vi "Actor Core.vi"(8 "error in":errorcluster, 11 "PRM in":refnum<class "PRM.lvclass">) -> (0 "error out":errorcluster, 3 "Actor out":refnum<class "Actor.lvclass">)   [LabVIEW 2019, in "PRM.lvlib" / "PRM.lvclass"]
doc: "The instrument actor core is only here to distribute panel resolution settings to children classes."
uses:
  Library/PRM.lvclass
  builds/Engine/Actor Framework.lvlibp/1abvi3w/vi.lib/ActorFramework/Actor/Actor.lvclass
  Custom Controls/Units.ctl
  PRM Messages/Set Channel by Name Msg/Set Channel by Name Msg.lvclass/Set Channel by Name Msg.ctl
  builds/Engine/Actor Framework.lvlibp/1abvi3w/vi.lib/ActorFramework/Message Enqueuer/Enqueue.vi
  PRM Messages/Set Channel by Name Msg/Set Channel by Name Msg.lvclass
  builds/Instruments/Instruments.lvlibp/Library/Instruments.lvclass
  C:/Users/Public/Documents/Development/builds/Instruments/Instruments.lvlibp/Library/Instruments.lvclass
panel:
  in  "Active Device":u16(ring)
  in  "Units":T1
  in  "Target":dbl caption="Ohms"
  in  "Active Channel":u16(ring) caption="Channel"
  in  "Apply":bool
  in  "Status":i32(listbox)
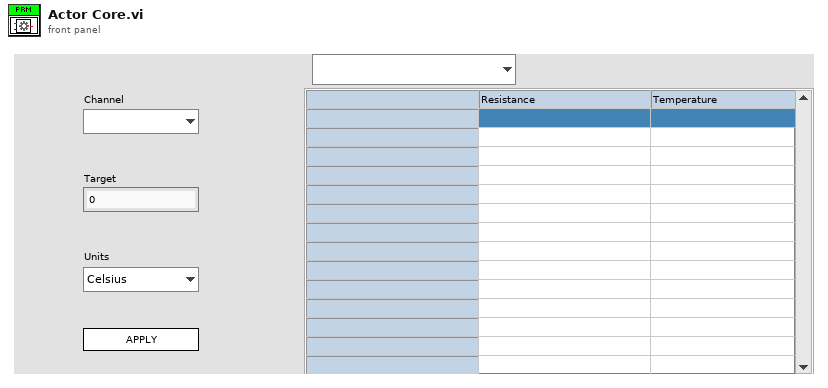
[diagram p1: front panel]
types:
  T1 = typedef "PRM.lvlib/PRM.lvclass/Units.ctl" = enum16{"Celsius", "Fahrenheit", "Kelvin", "Ohms"}
  T2 = cluster{"Pnl Actor":refnum<event-registration>, "Event Registration Refnum":refnum<event-registration>}
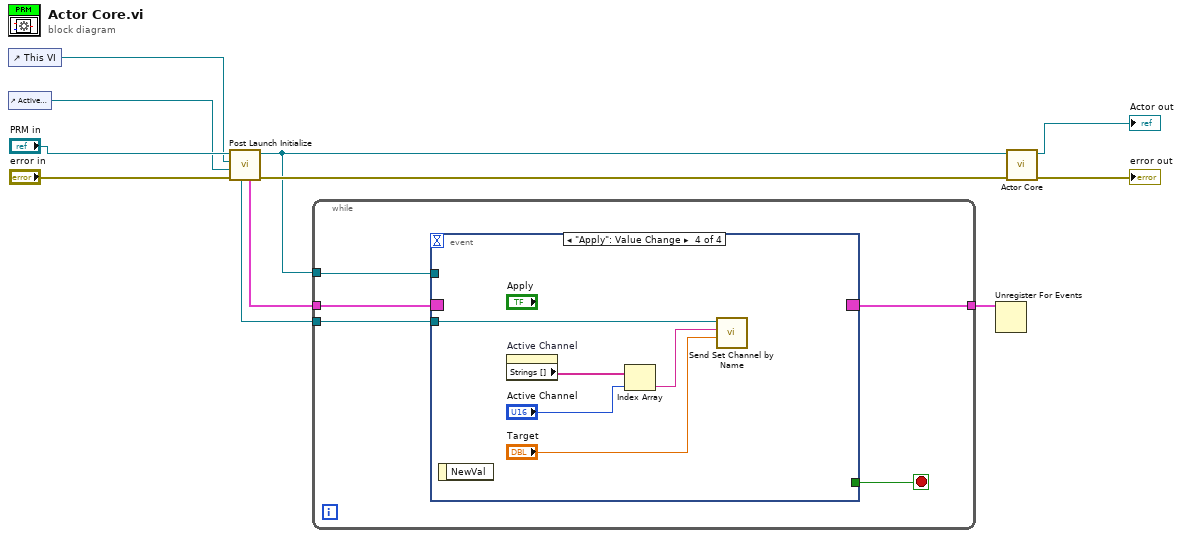
[diagram p0: block diagram]
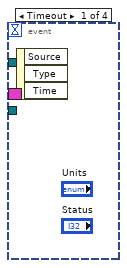
[diagram p2: hidden frame]
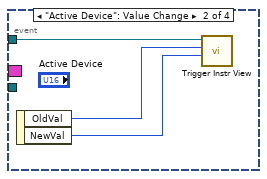
[diagram p3: hidden frame]
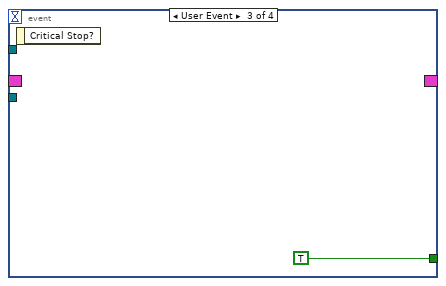
[diagram p4: hidden frame]
diagram:
  n1 = control-ref of="This VI"() -> (w2:refnum<vi>)
  n2 = control-ref of="Active Device"() -> (w1:refnum<vi>)
  n3 = call "Post Launch Initialize.vi"("error in"="error in", "Active Device"=w1, "GUI Reference"=w2, "Instruments in"="PRM in") -> ("error out"=w9:errorcluster, "Instruments out"=w6:refnum<class "PRM.lvclass">, "Registered Events"=w8:T2, "Self Enqueuer"=w7:refnum<class "Message Enqueuer.lvclass">)  [unwired: 4 in]
  n4 = while {
    tunnel: w8 -> [w16]
    tunnel: w7 -> [w15]
    tunnel: w6 -> [w14]
    tunnel: [w13] -> w5
    stop <- w12 stop-if-true
    n5 = event shown="[3] \"Apply\": Value Change" {
      selector: w16 -> [_ _ _ _]
      dyn-events: [_ _ _ _] -> w13
      timeout: _ -> [_ _ _ _]
      tunnel: w15 -> [_ _ _ w25]
      tunnel: w14 -> [_ w19 _ _]
      tunnel: [_ _ TRUE ("Discard?") _] -> w12
      event Timeout {
        n6 = event-data() -> ()  [unwired: 1 in, 3 out]
      }
      event "Active Device": Value Change {
        n7 = event-data() -> ("OldVal"=w18:u16, "NewVal"=w17:u16)  [unwired: 1 in]
        n8 = call "Trigger Instr View.vi"("New Value"=w17, "Old Value"=w18, "Instruments in"=w19) -> ()  [unwired: 7 in, 2 out]
      }
      event User Event {
        n9 = event-data() -> ()  [unwired: 1 in, 1 out]
      }
      event "Apply": Value Change {
        n10 = event-data() -> ()  [unwired: 1 in, 1 out]
        n11 = property on="Active Channel" class="Ring (strict)"() -> ("Strings []"=w24:string[])  [unwired: 2 in, 2 out]
        n12 = Index Array(array=w24, index="Active Channel") -> (element=w22:string)
        n13 = call "Send Set Channel by Name.vi"("Target"="Target", "Channel Name"=w22, "Message Enqueuer"=w25) -> ()  [unwired: 7 in, 2 out]
      }
    }
  }
  n14 = Unregister For Events(event registration refnum=w5) -> ()  [unwired: 1 in, 1 out]
  n15 = call-parent "Actor Core.vi"("error in"=w9, "Instruments in"=w6) -> ("error out"=→"error out":errorcluster, "Actor out"=→"Actor out":refnum<class "Actor.lvclass">)  [unwired: 8 in]
